vi "U6 Quadrature.vi"(8 "error in":errorcluster) -> (0 "error out":errorcluster)   [LabVIEW 2021]
panel:
  out "Pulses per Second":dbl format="%.2g"
  in  "Stop":bool
  in  "Reset Count":bool
  out "Quadrature Count":i32
  in  "FirstFound":bool=TRUE
  in  "Address":string="1"
  out "Error Message":string
  # "Demonstrates 1 quadrature input, which uses two timer channels for phases A and B (FIO0 and FIO1 in this case).\nIf you don't have a quadrature signal source handy, you can connect wires to GND, and tap these wires on FIO0\nand FIO1 to simulate quadrature."
  # "This VI passes a timer\nbase clock constant that\nis valid for hardware V1.21.\nFor hardware V1.20 change\nLJ_tc48MHZ to LJ_tc24MHZ."
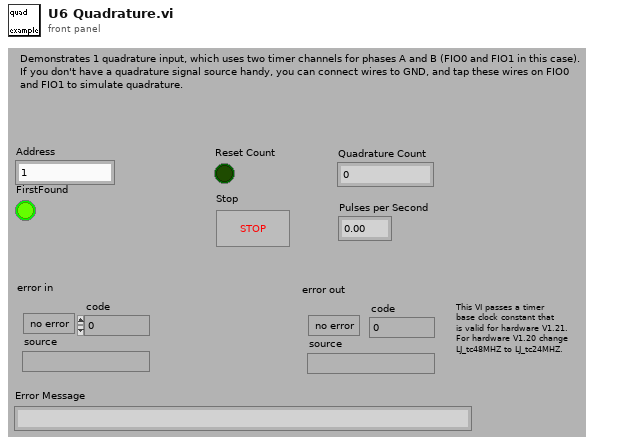
[diagram p1: front panel]
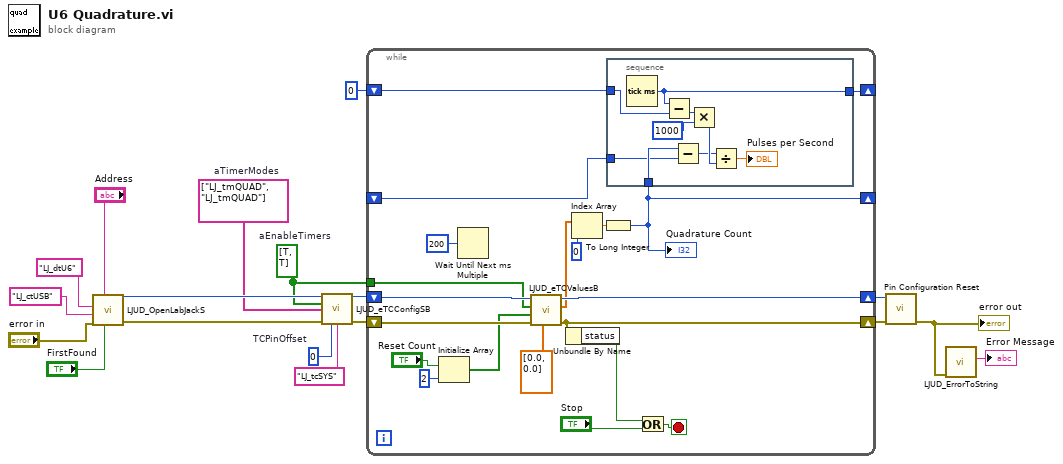
[diagram p0: block diagram]
diagram:
  w3 = 0  # TCPinOffset
  w2 = bool[] [TRUE, TRUE]  # aEnableTimers
  w5 = string[] ["LJ_tmQUAD", "LJ_tmQUAD"]  # aTimerModes
  n1 = call "LJUD_OpenLabJackS.vi"("FirstFound"="FirstFound", "Address"="Address", "error in"="error in", "ConnectionType"="LJ_ctUSB", "DeviceType"="LJ_dtU6") -> ("error out"=w9:errorcluster, "Handle"=w8:i32)  [unwired: 4 in, 1 out]
  n2 = call "LJUD_eTCConfigSB.vi"("Handle In"=w8, "aEnableTimers"=w2, "aTimerModes"=w5, "error in"=w9, "TCPinOffset"=w3, "TimerClockBase"="LJ_tcSYS") -> ("Handle Out"=w6:i32, "error out"=w7:errorcluster)  [unwired: 8 in]
  n3 = while {
    tunnel: w2 -> [w25]
    shift-left: w7 -> [w27]
    shift-right: [w37] -> w11
    shift-left: w6 -> [w28]
    shift-right: [w30] -> w12
    shift-right: [w23] -> _
    shift-left: u32 0 ("millisecond timer value") -> [w22]
    shift-right: [w20] -> _
    shift-left: _ -> [w19]
    stop <- w36 stop-if-true
    n4 = Initialize Array("Reset Count", 2 ("Dimension Size")) -> (w24:bool[])
    n5 = Wait Until Next ms Multiple(millisecond multiple=u32 200) -> ()  [unwired: 1 out]
    n6 = call "LJUD_eTCValuesB.vi"("aTimerValues Write"=dbl[] [0.0, 0.0], "error in"=w27, "aUpdateResetTimers"=w24, "aReadTimers"=w25, "Handle In"=w28) -> ("error out"=w37:errorcluster, "aTimerValues Read"=w29:dbl[], "Handle Out"=w30:i32)  [unwired: 3 in, 1 out]
    n7 = Unbundle By Name(w37) -> ("status"=w35:bool)
    n8 = Index Array(array=w29, index=0 ("Index")) -> (element=w21:dbl)
    n9 = To Long Integer(number=w21) -> (32bit integer=w20:i32)
    "Quadrature Count" <- w20
    n10 = stacked-sequence {
      tunnel: [w47] -> w23
      tunnel: w22 -> [w46]
      tunnel: w20 -> [w42]
      tunnel: w19 -> [w41]
      frame #0 {
        n11 = Tick Count (ms)() -> (millisecond timer value=w47:u32)
        n12 = Subtract(x=w47, y=w46) -> (x-y=w45:u32)
        n13 = Subtract(x=w42, y=w41) -> (x-y=w40:i32)
        n14 = Multiply(x=w45, y=u32 1000) -> (x*y=w44:u32)
        n15 = Divide(x=w40, y=w44) -> (x/y=→"Pulses per Second":dbl)
      }
    }
    n16 = Or(x=w35, y="Stop") -> (x .or. y?=w36:bool)
  }
  n17 = call "Pin Configuration Reset.vi"("error in"=w11, "Handle In"=w12) -> ("error out"=w10:errorcluster)  [unwired: 8 in, 1 out]
  "error out" <- w10
  n18 = call "LJUD_ErrorToString.vi"("error in"=w10) -> ("String"=→"Error Message":string)  [unwired: 10 in]
